vi "Sub_Set_Voltage_Output.vi"(0 "AgB29xxLib.IAgB29xx2":refnum<k7>, 5 "i":i32, 7 "Level":dbl=20.0, 9 "Range":dbl=2.0, 11 "error in":errorcluster, 12 "AutoRangeEnabled":bool, 13 "TriggeredLevel":dbl=2.0, 14 "RangeLowerLimit":dbl) -> (4 "AgB29xxLib.IAgB29xx2 2":refnum<k7>, 15 "error out":errorcluster)   [LabVIEW 2009]
panel:
  # "SubVI: Set Voltage Output"
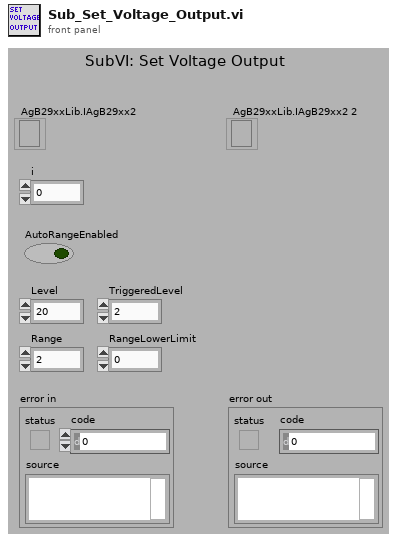
[diagram p1: front panel]
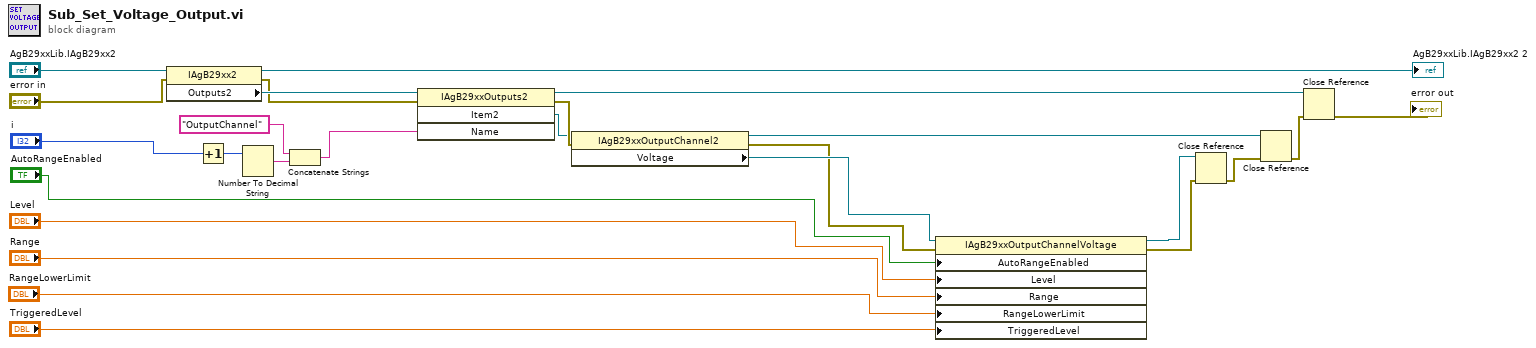
[diagram p0: block diagram]
diagram:
  n1 = property class="IAgB29xx2"(reference="AgB29xxLib.IAgB29xx2", error in="error in") -> (reference out=→"AgB29xxLib.IAgB29xx2 2":refnum<k7>, error out=w1:errorcluster, "Outputs2"=w23:refnum<k7>)
  n2 = Increment(x="i") -> (x+1=w22:i32)
  n3 = Number To Decimal String(number=w22) -> (decimal integer string=w21:string)  [unwired: 1 in]
  n4 = Concatenate Strings("OutputChannel" ("string"), w21) -> (w19:string)
  n5 = invoke class="IAgB29xxOutputs2" method="Item2"(reference=w23, error in=w1, "Name"=w19) -> (reference out=w14:refnum<k7>, error out=w18:errorcluster, "Item2"=w12:refnum<k7>)  [unwired: 1 in, 1 out]
  n6 = property class="IAgB29xxOutputChannel2"(reference=w12, error in=w18) -> (reference out=w16:refnum<k7>, error out=w6:errorcluster, "Voltage"=w7:refnum<k7>)
  n7 = property class="IAgB29xxOutputChannelVoltage"(reference=w7, error in=w6, "AutoRangeEnabled"="AutoRangeEnabled", "Level"="Level", "Range"="Range", "RangeLowerLimit"="RangeLowerLimit", "TriggeredLevel"="TriggeredLevel") -> (reference out=w3:refnum<k7>, error out=w4:errorcluster)
  n8 = Close Reference(reference=w3, error in (no error)=w4) -> (error out=w17:errorcluster)
  n9 = Close Reference(reference=w16, error in (no error)=w17) -> (error out=w15:errorcluster)
  n10 = Close Reference(reference=w14, error in (no error)=w15) -> (error out=→"error out":errorcluster)
